vi "Run.vi"(8 "error in (no error)":errorcluster, 9 "s on last turn":dbl, 10 "Maze (0: Empty, -1: Enemy. >0: Teammate":i32[][](array[numeric])=[[16, 0, 18], [0, 14, 0], [0, 0, 0]], 11 "Borg In":refnum<class "Borg.lvclass">) -> (0 "error out":errorcluster, 1 "Direction":T1, 2 "Action":T2, 3 "Borg Out":refnum<class "Borg.lvclass">, 4 "Replicated":refnum<class "Square.lvclass">)   [LabVIEW 2015, in "Borg.lvclass"]
uses:
  Borg.lvclass
  Type Defs/Action Enum.ctl
  Type Defs/Direction Enum.ctl
  Square/Square.lvclass
  Type Defs/SB Type Defs.lvlib
  Common/Common.lvlib
panel:
  in  "Status":string
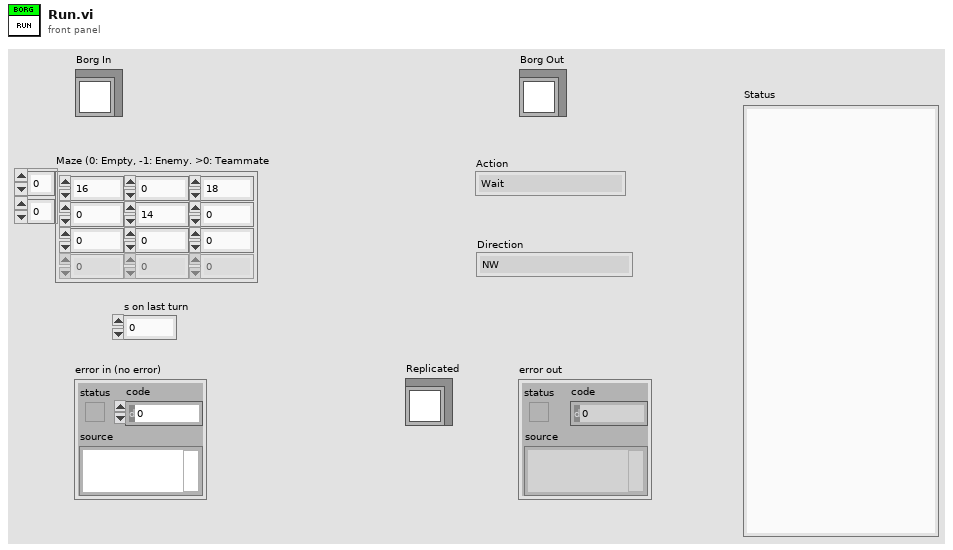
[diagram p1: front panel]
types:
  T1 = typedef "SB Type Defs.lvlib/Direction Enum.ctl" = enum16{"NW", "N", "NE", "E", "SE", "S", "SW", "W"}
  T2 = typedef "SB Type Defs.lvlib/Action Enum.ctl" = enum16{"Wait", "Move", "Attack", "Replicate"}
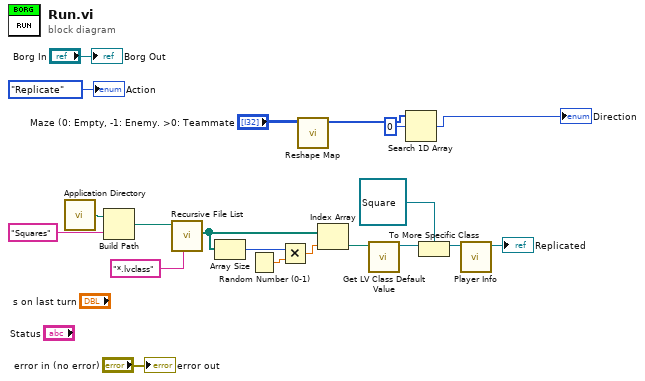
[diagram p0: block diagram]
diagram:
  n1 = call <vilib>:"Application Directory.vi"() -> ("Application Directory"=w13:path)
  n2 = Build Path(base path=w13, name or relative path="Squares") -> (appended path=w15:path)
  n3 = call <vilib>:"Recursive File List.vi"("pattern"="*.lvclass", "Folder Path"=w15) -> ("All Files in Dir"=w8:path[])  [unwired: 5 in, 4 out]
  n4 = Array Size(array=w8) -> (size(s)=w10:i32)
  n5 = Random Number (0-1)() -> (number: 0 to 1=w11:dbl)
  n6 = Multiply(x=w10, y=w11) -> (x*y=w6:dbl)
  n7 = call "Reshape Map.vi"("Maze (0: Empty, -1: Enemy. >0: Teammate"="Maze (0: Empty, -1: Enemy. >0: Teammate") -> ("Map"=w3:i32[])  [unwired: 9 in, 1 out]
  n8 = Index Array(array=w8, index=w6) -> (element=w7:path)
  n9 = call <vilib>:"Get LV Class Default Value.vi"("class path"=w7) -> ("object"=w16:refnum<class>)  [unwired: 9 in, 1 out]
  n10 = Search 1D Array(1D array=w3, element=0) -> (index of element=→"Direction":i32)  [unwired: 1 in]
  n11 = To More Specific Class(target class=refnum<class "Square.lvclass"> refnum ("Runner.lvclass"), reference=w16) -> (specific class reference=w18:refnum<class "Square.lvclass">)  [unwired: 1 in, 1 out]
  n12 = call-dynamic "Player Info.vi"("Square in"=w18) -> ("Square out"=→"Replicated":refnum<class "Square.lvclass">)  [unwired: 8 in, 2 out]
  "error out" <- "error in (no error)"
  "Borg Out" <- "Borg In"
  "Action" <- Action_Enum."Replicate" ("Action")
